vi "Shooter Solenoid Refnums fg.vi"() -> ()   [LabVIEW 2013]
uses:
  <vilib>/Rock Robotics/WPI/Solenoid/WPI_SolenoidDevRef.ctl
  <vilib>/Rock Robotics/SystemInterfaces/Typedef/FPGA_TypedefSolenoidModule.ctl
  <vilib>/Rock Robotics/WPI/Solenoid/WPI_SolenoidChannel.ctl
  <vilib>/Rock Robotics/WPI/DigitalInput/WPI_DigitalInputDevRef.ctl
  <vilib>/Rock Robotics/SystemInterfaces/DIO/FPGA_DIOChannel.ctl
  <vilib>/Rock Robotics/SystemInterfaces/Typedef/FPGA_TypedefDigitalModule.ctl
  UberCode 2-18-14/typedefs/fg_typedef.ctl
panel:
  in  "Menu":T1
  out "Right Down DevRef 2":T2
  out "Right Up DevRef 2":T2
  out "Latch Solenoid DevRef 2":T5={"DevStatus"={"status"=FALSE, "code"=0, "source"=""}, "Solenoid Module"=enum."Solenoid Module 1", "Forward Solenoid Channel"=enum."Invalid", "Reverse Solenoid Channel"=enum."Invalid"}
  out "Shooter Solenoid DevRef 2":T5={"DevStatus"={"status"=FALSE, "code"=0, "source"=""}, "Solenoid Module"=enum."Solenoid Module 1", "Forward Solenoid Channel"=enum."Invalid", "Reverse Solenoid Channel"=enum."Invalid"}
  in  "Right Down DevRef":T2={"DevStatus"={"status"=FALSE, "code"=0, "source"=""}, "DIO Channel"=enum."Invalid", "Digital Module"=enum."Digital Module 1"}
  in  "Right Up DevRef":T2={"DevStatus"={"status"=FALSE, "code"=0, "source"=""}, "DIO Channel"=enum."Invalid", "Digital Module"=enum."Digital Module 1"}
  in  "Latch Solenoid DevRef":T5={"DevStatus"={"status"=FALSE, "code"=0, "source"=""}, "Solenoid Module"=enum."Solenoid Module 1", "Forward Solenoid Channel"=enum."Invalid", "Reverse Solenoid Channel"=enum."Invalid"}
  in  "Shooter Solenoid DevRef":T5={"DevStatus"={"status"=FALSE, "code"=0, "source"=""}, "Solenoid Module"=enum."Solenoid Module 1", "Forward Solenoid Channel"=enum."Invalid", "Reverse Solenoid Channel"=enum."Invalid"}
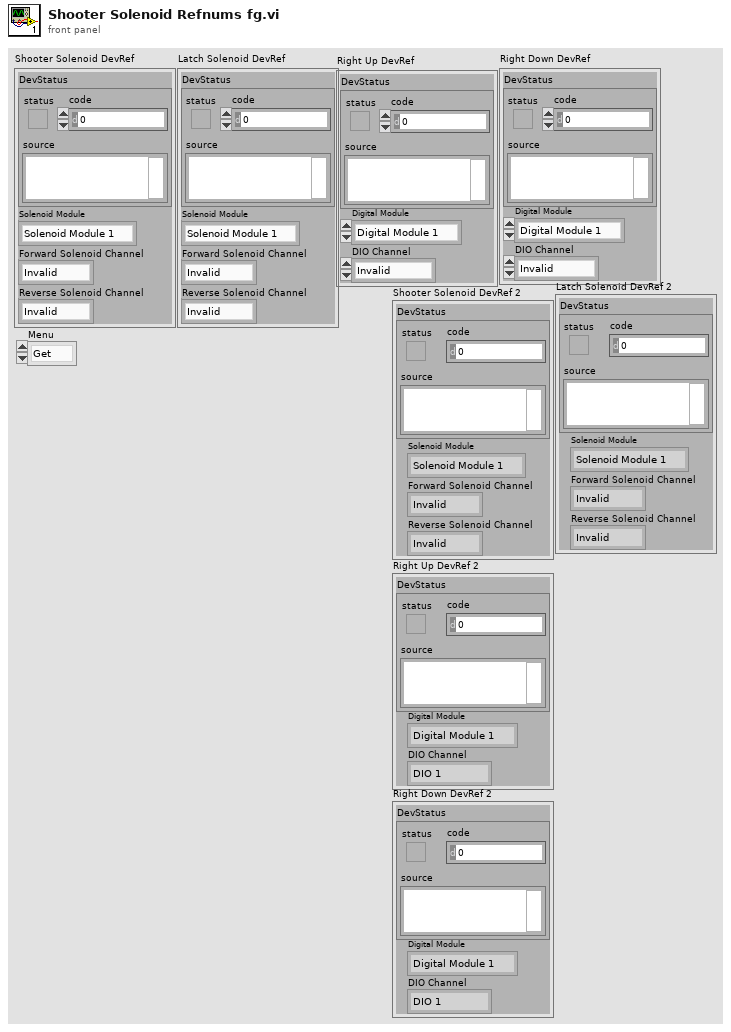
[diagram p1: front panel]
types:
  T1 = typedef "fg_typedef.ctl" = enum16{"Get", "Set"}
  T2 = typedef "WPI_DigitalInputDevRef.ctl" = cluster{"DevStatus":errorcluster, "DIO Channel":T3, "Digital Module":T4}
  T3 = typedef "FPGA_DIOChannel.ctl" = enum8{"DIO 1", "DIO 2", "DIO 3", "DIO 4", "DIO 5", "DIO 6", "DIO 7", "DIO 8", "DIO 9", "DIO 10", "DIO 11", "DIO 12", "DIO 13", "DIO 14", "Invalid"}
  T4 = typedef "FPGA_TypedefDigitalModule.ctl" = enum16{"Digital Module 1", "Digital Module 2"}
  T5 = typedef "WPI_SolenoidDevRef.ctl" = cluster{"DevStatus":errorcluster, "Solenoid Module":T6, "Forward Solenoid Channel":T7, "Reverse Solenoid Channel":T7}
  T6 = typedef "FPGA_TypedefSolenoidModule.ctl" = enum16{"Solenoid Module 1", "Solenoid Module 2"}
  T7 = typedef "WPI_SolenoidChannel.ctl" = enum8{"Solenoid 1", "Solenoid 2", "Solenoid 3", "Solenoid 4", "Solenoid 5", "Solenoid 6", "Solenoid 7", "Solenoid 8", "Invalid"}
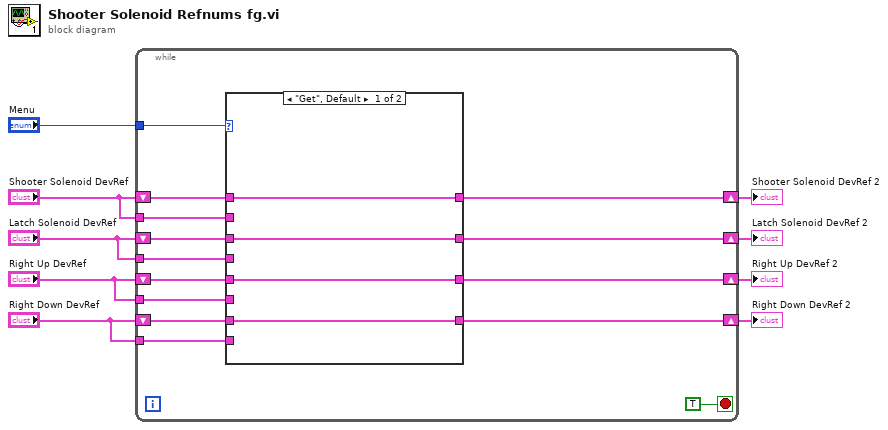
[diagram p0: block diagram]
diagram:
  n1 = while {
    shift-right: [w17] -> w9
    shift-left: "Shooter Solenoid DevRef" -> [w22]
    shift-right: [w16] -> w8
    shift-left: "Latch Solenoid DevRef" -> [w21]
    shift-right: [w15] -> w7
    shift-left: "Right Up DevRef" -> [w19]
    shift-right: [w14] -> w6
    shift-left: "Right Down DevRef" -> [w18]
    tunnel: "Menu" -> [w20]
    tunnel: "Shooter Solenoid DevRef" -> [w13]
    tunnel: "Latch Solenoid DevRef" -> [w12]
    tunnel: "Right Up DevRef" -> [w11]
    tunnel: "Right Down DevRef" -> [w10]
    stop <- TRUE stop-if-true
    n2 = case shown="\"Get\", Default" w20 {
      tunnel: w22 -> [w27 _]
      tunnel: w21 -> [w26 _]
      tunnel: w19 -> [w25 _]
      tunnel: w18 -> [w24 _]
      tunnel: [w27 w31] -> w17
      tunnel: [w26 w30] -> w16
      tunnel: [w25 w29] -> w15
      tunnel: [w24 w28] -> w14
      tunnel: w13 -> [_ w31]
      tunnel: w12 -> [_ w30]
      tunnel: w11 -> [_ w29]
      tunnel: w10 -> [_ w28]
      frame "Get", Default {
      }
      frame "Set" {
      }
    }
  }
  "Shooter Solenoid DevRef 2" <- w9
  "Latch Solenoid DevRef 2" <- w8
  "Right Up DevRef 2" <- w7
  "Right Down DevRef 2" <- w6
